vi "timer test.vi"() -> ()   [LabVIEW 2010]
uses:
  timer control.ctl
panel:
  in  "Data Entry Limits:Maximum":dbl
  out "Thermometer":dbl(slide) max=80.0 scale=0.0..87.0
  out "Array":string[](array[string])
  in  "timer":T1={"Thermometer"=0.0, "last check (sec)"=nan, "interval (sec)"=nan, "type"=enum."countdown"} {"Thermometer" scale=0.0..87.0}
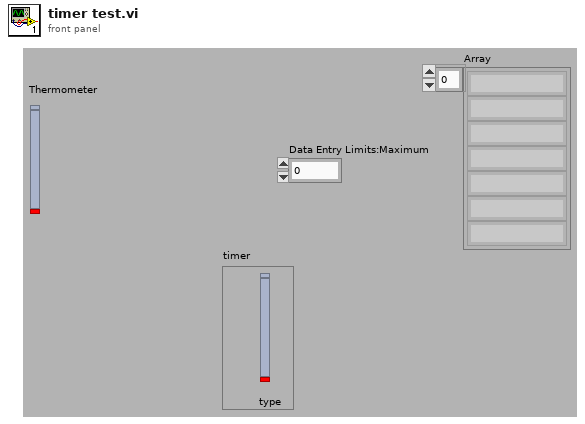
[diagram p1: front panel]
types:
  T1 = typedef "timer control.ctl" = cluster{"Thermometer":dbl, "last check (sec)":dbl, "interval (sec)":dbl, "type":enum16{"countdown", "periodic", ""}}
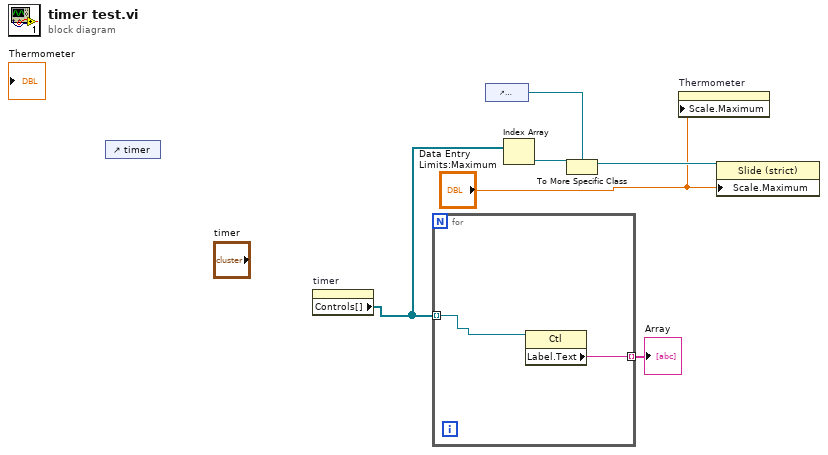
[diagram p0: block diagram]
diagram:
  n1 = control-ref of="timer"() -> ()  [unwired: 1 out]
  n2 = property on="timer" class="Clust (strict)"() -> ("Controls[]"=w5:refnum<vi>[])  [unwired: 2 in, 2 out]
  n3 = for {
    tunnel: w5 -> [w8] mode=indexing
    tunnel: [w7] -> w6 mode=indexing
    n4 = property class="Ctl"(reference=w8) -> ("Label.Text"=w7:string)  [unwired: 1 in, 2 out]
  }
  "Array" <- w6
  n5 = control-ref of="Thermometer"() -> (w3:refnum<vi>)
  n6 = Index Array(array=w5) -> (element=w4:refnum<vi>)  [unwired: 1 in]
  n7 = To More Specific Class(target class=w3, reference=w4) -> (specific class reference=w2:refnum<vi>)  [unwired: 1 in, 1 out]
  n8 = property on="Thermometer" class="Slide (strict)"("Scale.Maximum"="Data Entry Limits:Maximum") -> ()  [unwired: 2 in, 2 out]
  n9 = property class="Slide (strict)"(reference=w2, "Scale.Maximum"="Data Entry Limits:Maximum") -> ()  [unwired: 1 in, 2 out]
